vi "Preview Single D2Binary.vi"(8 "Error In":errorcluster, 9 "Boolean index":i32, 10 "D index":i32, 11 "Queue in":refnum<queue>) -> (0 "Error Out":errorcluster, 1 "element":bool, 3 "SEQ out":refnum<queue>)   [LabVIEW 2019, in "FX5U SLMP Binary.lvlib"]
uses:
  FX5U SLMP Binary.lvlib
  Data Cluster.ctl
panel:
  out "D value":i16
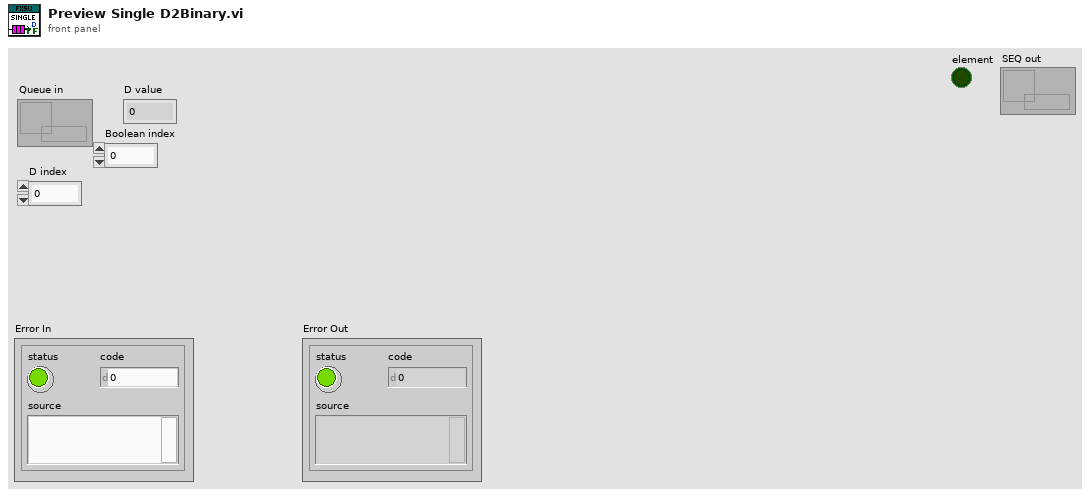
[diagram p1: front panel]
types:
  T1 = typedef "FX5U SLMP Binary.lvlib/Data Cluster.ctl" = cluster{"M Array":bool[], "D Array":i16[]}
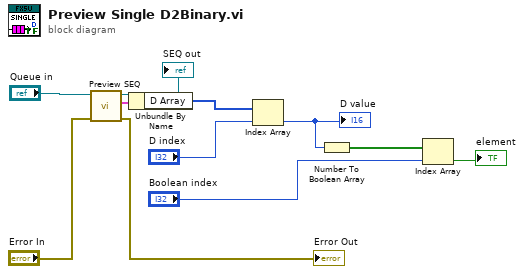
[diagram p0: block diagram]
diagram:
  n1 = call "Preview SEQ.vi"("Error In"="Error In", "SEQ in"="Queue in") -> ("Error Out"=→"Error Out":errorcluster, "Data Cluster"=w8:T1, "SEQ out"=→"SEQ out":refnum<queue>)  [unwired: 7 in]
  n2 = Unbundle By Name(w8) -> ("D Array"=w9:i16[])
  n3 = Index Array(array=w9, index="D index") -> (element=w5:i16)
  "D value" <- w5
  n4 = Number To Boolean Array(number=w5) -> (Boolean array=w4:bool[])
  n5 = Index Array(array=w4, index="Boolean index") -> (element=→"element":bool)
